vi "Set_MultiVar_BulkMode_Values.vi"(8 "error in (no error)":errorcluster, 9 "varValues":dbl[][](array[numeric]) format="%#_13g", 10 "varNames":string[](array[string]), 11 "mupExpr in":refnum<data-value>) -> (0 "error out":errorcluster, 3 "mupExpr out":refnum<data-value>)   [LabVIEW 2015, in "mupExpr.lvclass"]
doc: "Set the bulk mode values for a list of variables.\n\nNote that the array of values provided for variable values should be of size:\nNum Rows: Number of Variables\nNum Cols: Bulk Size\n\nIf any variable is not found, a warning is generated."
uses:
  mupExpr.lvclass
  mupExpr.lvclass/mupExpr.ctl
  mupLib/mupSetVarValue_Array.vi
  <vilib>/Utility/error.llb/Error Cluster From Error Code.vi
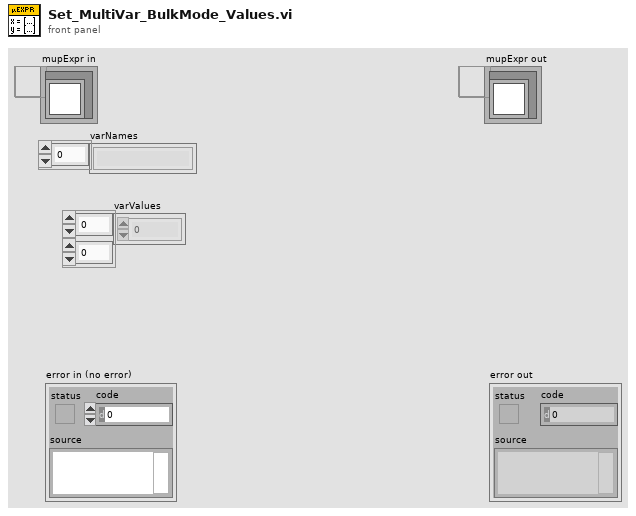
[diagram p1: front panel]
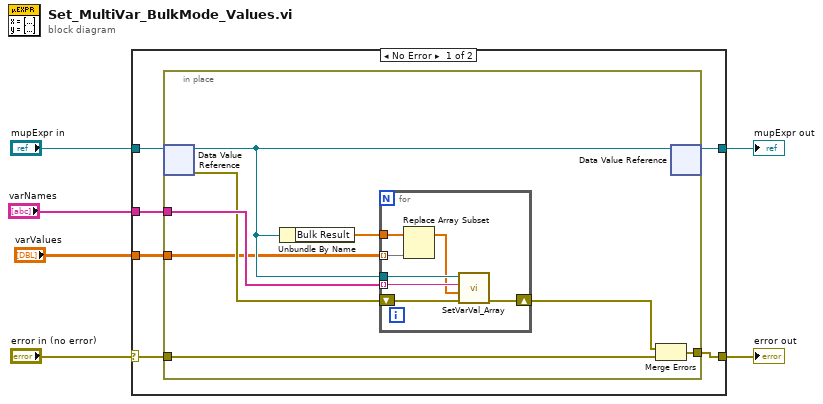
[diagram p0: block diagram]
diagram:
  n1 = case shown="No Error" "error in (no error)" {
    selector: "error in (no error)" -> [w7 w28]
    tunnel: "varValues" -> [w12 _]
    tunnel: "varNames" -> [w11 _]
    tunnel: "mupExpr in" -> [w10 w29]
    tunnel: [w9 w28] -> w3
    tunnel: [w8 w29] -> w2
    frame No Error {
      n2 = in-place {
        in-place-border: w7 -> [w17]
        in-place-border: w12 -> [w13]
        in-place-border: w11 -> [w20]
        in-place-border: [w16] -> w9
        n3 = in-place-dvr #1(w10) -> (w15:refnum<class "mupExpr.lvclass">, w19:errorcluster)
        n4 = Unbundle By Name(w15) -> ("Bulk Result"=w14:dbl[])
        n5 = for {
          tunnel: w20 -> [w27] mode=indexing
          tunnel: w15 -> [w24]
          tunnel: w14 -> [w23]
          tunnel: w13 -> [w22] mode=indexing
          shift-right: [w25] -> w18
          shift-left: w19 -> [w26]
          n6 = Replace Array Subset(array=w23, new element=w22) -> (w21:dbl[])  [unwired: 1 in]
          n7 = call "SetVarVal_Array.vi"("error in (no error)"=w26, "varValue"=w21, "varName"=w27, "muExpr in"=w24) -> ("error out"=w25:errorcluster)  [unwired: 6 in, 1 out]
        }
        n8 = Merge Errors(w18, w17) -> (w16:errorcluster)
        n9 = in-place-dvr #1(w15) -> (w8:refnum<data-value>)  [unwired: 1 out]
      }
    }
    frame Error {
    }
  }
  "error out" <- w3
  "mupExpr out" <- w2
